vi "rename seq channel in mappings.vi"(8 "error in":errorcluster, 9 "new seq channel name":string, 10 "old seq channel name":string, 11 "engine configuration in":refnum<class "base TBM sequencer configuration.lvclass">) -> (0 "error out":errorcluster, 3 "engine configuration out":refnum<class "base TBM sequencer configuration.lvclass">)   [LabVIEW 2014, in "base TBM sequencer configuration.lvclass"]
uses:
  base TBM sequencer configuration.lvclass
  base TBM sequencer configuration.lvclass/base TBM sequencer configuration.ctl
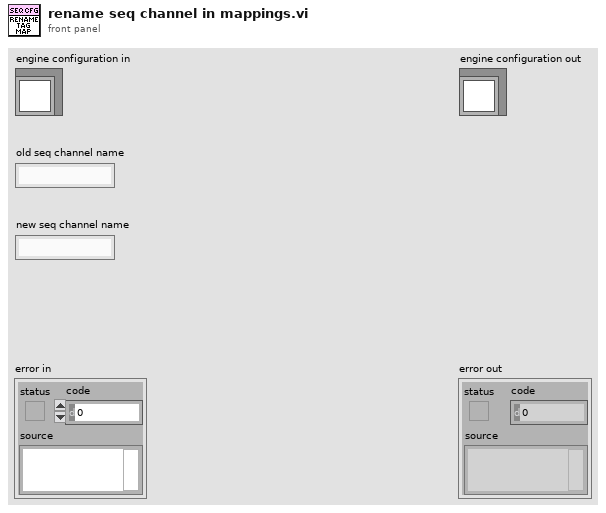
[diagram p1: front panel]
types:
  T1 = typedef "base TBM sequencer configuration.lvclass/Module Mappings.ctl" = cluster{"Owning ID":string, "Input Mappings":T2[], "Process Parameter Mappings":T2[], "Process Results Mappings":T2[], "Output Mappings":T2[]}
  T2 = typedef "tag bus.lvlib/data table.lvlib/mapping specification.ctl" = cluster{"data type":T3, "mappings":T4[]}
  T3 = typedef "tag bus.lvlib/tag descriptor.lvclass/Data Type.ctl" = enum16{"Double", "Single", "I64", "I32", "I16", "I8", "U64", "U32", "U16", "U8", "Boolean", "String", "Array of Double", "Array of Single", "Array of I64", "Array of I32", "Array of I16", "Array of I8", "Array of U64", "Array of U32", "Array of U16", "Array of U8", "Array of Boolean", "Array of String"}
  T4 = typedef "tag bus.lvlib/data table.lvlib/mapping.ctl" = cluster{"sink name":string, "source name":string}
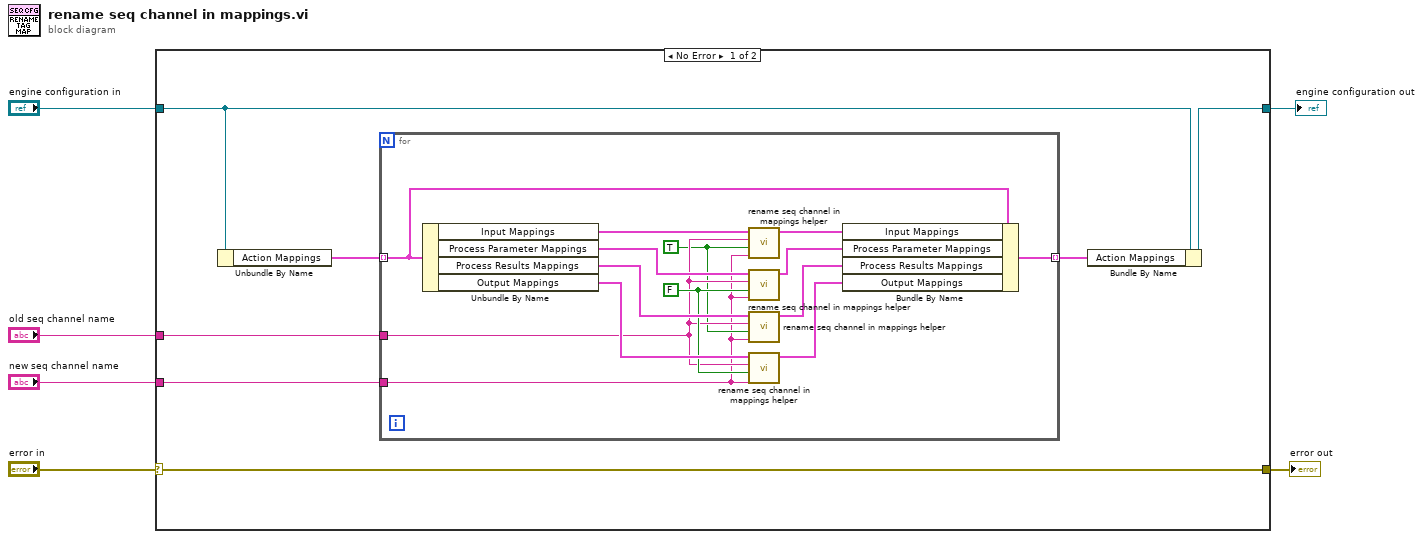
[diagram p0: block diagram]
diagram:
  n1 = case shown="No Error" "error in" {
    selector: "error in" -> [w13 w29]
    tunnel: [w13 w29] -> w2
    tunnel: [w8 w28] -> w3
    tunnel: "engine configuration in" -> [w10 w28]
    tunnel: "old seq channel name" -> [w12 _]
    tunnel: "new seq channel name" -> [w7 _]
    frame No Error {
      n2 = Unbundle By Name(w10) -> ("Action Mappings"=w11:T1[])
      n3 = for {
        tunnel: w12 -> [w22]
        tunnel: w11 -> [w21] mode=indexing
        tunnel: [w16] -> w9 mode=indexing
        tunnel: w7 -> [w14]
        w23 = FALSE
        w15 = TRUE
        n4 = Unbundle By Name(w21) -> ("Input Mappings"=w27:T2[], "Process Parameter Mappings"=w26:T2[], "Process Results Mappings"=w25:T2[], "Output Mappings"=w24:T2[])
        n5 = call "rename seq channel in mappings helper.vi"("new seq channel name"=w14, "input channel?"=w15, "old seq channel name"=w22, "Mappings"=w27) -> ("Mappings out"=w20:T2[])  [unwired: 7 in]
        n6 = call "rename seq channel in mappings helper.vi"("new seq channel name"=w14, "input channel?"=w23, "old seq channel name"=w22, "Mappings"=w26) -> ("Mappings out"=w19:T2[])  [unwired: 7 in]
        n7 = call "rename seq channel in mappings helper.vi"("new seq channel name"=w14, "input channel?"=w15, "old seq channel name"=w22, "Mappings"=w25) -> ("Mappings out"=w18:T2[])  [unwired: 7 in]
        n8 = call "rename seq channel in mappings helper.vi"("new seq channel name"=w14, "input channel?"=w23, "old seq channel name"=w22, "Mappings"=w24) -> ("Mappings out"=w17:T2[])  [unwired: 7 in]
        n9 = Bundle By Name(cluster=w21, "Input Mappings"=w20, "Process Parameter Mappings"=w19, "Process Results Mappings"=w18, "Output Mappings"=w17) -> (w16:T1)
      }
      n10 = Bundle By Name(cluster=w10, "Action Mappings"=w9) -> (w8:refnum<class "base TBM sequencer configuration.lvclass">)
    }
    frame Error {
    }
  }
  "error out" <- w2
  "engine configuration out" <- w3
